vi "ProcessModbusUpdates.vi"(11 "MockFAILCSettings":T1={"ModbusRxDataFIFO"="ModbusSubnetARxDataFIFO", "ModbusTxDataFIFO"="ModbusSubnetATxDataFIFO", "BufferUpdateFIFO"="MockFAILC1Command", "Code17Memory"="MockFAILC1Code17", "Code18Memory"="MockFAILC1Code18", "Code65Memory"="MockFAILC1Code65", "Code72Memory"="MockFAILC1Code72", "Code74Memory"="MockFAILC1Code74", "Code75Memory"="MockFAILC1Code75", "Code76Memory"="MockFAILC1Code76", "Code80Memory"="MockFAILC1Code80", "Code110Memory"="MockFAILC1Code110", "Code120Memory"="MockFAILC1Code120", "Code121Memory"="MockFAILC1Code121", "CRCDataFIFO"="MockFAILC1CRCDataFIFO", "CRCCalculateFIFO"="MockFAILC1CRCCalculateFIFO", "CRCFIFO"="MockFAILC1CRCFIFO"}) -> ()   [LabVIEW 2016, in "FPGAMockFAILC.lvlib"]
uses:
  FPGAMockFAILC.lvlib
  DataTypes/MockFAILCSettings.ctl
  FPGAMockHPILC/DataTypes/MockHPModbusUpdateLoopData.ctl
  FPGAMockHPILC/DataTypes/MockHPModbusUpdateStates.ctl
  <vilib>/Platform/TimedLoop/XDataNode/timing_clust.ctl
  <vilib>/Platform/TimedLoop/XDataNode/nitl_modes.ctl
  <vilib>/Platform/TimedLoop/XDataNode/wakeup.ctl
  <vilib>/rvi/Emulation/niFpgaSctlEmulationGetInTimedLoop.vi
  <vilib>/rvi/Emulation/niFpgaEmulationReportErrorSimple.vi
  <vilib>/rvi/Emulation/niFpgaGetClockAttributes.vi
  <vilib>/rvi/Emulation/niFpgaCriticalErrorInLSC.vi
  <vilib>/rvi/DataTransferAndStorage/Container/Common/niFpgaContainerExecOnDevCompGetState.vi
  <vilib>/rvi/Emulation/niFpgaEmulationIsFPGAContextNoSignature.vi
  <vilib>/rvi/errors/niFpgaSetErrorForExecOnDevCompSimple.vi
  <vilib>/rvi/eio/common/nirviEmuReportErrorAndStop.vi
  <vilib>/rvi/DataTransferAndStorage/Container/Common/niFpgaContainerGetUniqueNameForEmu.vi
  <vilib>/rvi/FIFO/Fifo_Resource/nirvififoEmulationSetSize.vi
  <vilib>/rvi/FIFO/Fifo_Resource/nirviFifoEmulationQueueMgr.vi
  <instcachedir>/0/nirviFifoEmulationQueueMgr_E5CAEC123FF24DC58D834DCA3CDAA9B5.lvgen/nirviFifoEmulationQueueMgr_E5CAEC123FF24DC58D834DCA3CDAA9B5_002.vi
  <vilib>/rvi/FIFO/Fifo_Resource/nirvififoEmulationDetermineInputValidOut.vi
  <vilib>/rvi/FIFO/Fifo_Resource/nirvififoEmulationCreateLock.vi
  <vilib>/rvi/Emulation/niFpgaProcessEmulError.vi
  <vilib>/rvi/FIFO/Fifo_Resource/nirvififoEmulationObtainLock.vi
  <vilib>/rvi/FIFO/Fifo_Resource/nirvififoEmulationReleaseLock.vi
  <vilib>/rvi/occurrence/nirviWaitOnOccurrenceBase.vi
  <vilib>/rvi/errors/nirviReportUnexpectedCaseInternalError.vi
  <vilib>/rvi/errors/nirviReportUnexpectedCaseInternalError (U32).vi
  <vilib>/Utility/error.llb/Clear Errors.vi
  <vilib>/rvi/interface/RandomDataEmulation/niFpgaRandomDataHandleErrors.vi
  <instcachedir>/0/nirviFifoEmulationQueueMgr_E5CAEC123FF24DC58D834DCA3CDAA9B5.lvgen/nirviFifoEmulationQueueMgr_E5CAEC123FF24DC58D834DCA3CDAA9B5_000.vi
  <vilib>/rvi/Memory/Memory_Emulation/niFpgaMemoryEmulationCacheClearOnFirstRun.vi
  <vilib>/rvi/Memory/Memory_Emulation/nirvimemoryEmulationManagerCache_MakeExclusive.vi
  <vilib>/rvi/Memory/Memory_Emulation/niFpgaMemoryEmulationValidateCache.vi
  <vilib>/rvi/Memory/Memory_Emulation/nirvimemoryEmulationManagerCache_InsertValue.vi
  <vilib>/rvi/Memory/Memory_Emulation/nirvimemoryEmulationManagerCache_ReleaseExclusive.vi
  <vilib>/rvi/Memory/Memory_Emulation/nirvimemoryEmulationManagerCache_GetValue.vi
  <vilib>/rvi/Memory/Memory_Emulation/nirvimemoryEmulationManagerCache_SetValue.vi
  <vilib>/rvi/Emulation/niFpgaSctlEmulationResourceMgr.vi
  <instcachedir>/0/nirviFifoEmulationQueueMgr_E5CAEC123FF24DC58D834DCA3CDAA9B5.lvgen/nirviFifoEmulationQueueMgr_E5CAEC123FF24DC58D834DCA3CDAA9B5_001.vi
  <vilib>/Platform/TimedLoop/XDataNode/XDataNode.xnode
  <vilib>/rvi/DataTransferAndStorage/Container/XNode/niFpgaContainer.xnode
  <vilib>/rvi/FIFO/Fifo_Resource/niFpgaFifoEmulationRefIn.vi
  <vilib>/rvi/Memory/Memory_Emulation/niFpgaMemoryEmulationRefIn.vi
  FPGAMockHPILC/FPGAMockHPILC.lvlib
  <vilib>/Platform/TimedLoop/XDataNode/XDNodeRunTimeDep.lvlib
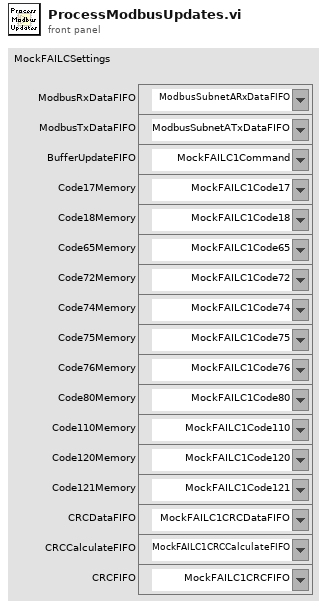
[diagram p1: front panel]
types:
  T1 = typedef "FPGAMockFAILC.lvlib/MockFAILCSettings.ctl" = cluster{"ModbusRxDataFIFO":refnum<k21>, "ModbusTxDataFIFO":refnum<k21>, "BufferUpdateFIFO":refnum<k21>, "Code17Memory":refnum<k21>, "Code18Memory":refnum<k21>, "Code65Memory":refnum<k21>, "Code72Memory":refnum<k21>, "Code74Memory":refnum<k21>, "Code75Memory":refnum<k21>, "Code76Memory":refnum<k21>, "Code80Memory":refnum<k21>, "Code110Memory":refnum<k21>, "Code120Memory":refnum<k21>, "Code121Memory":refnum<k21>, "CRCDataFIFO":refnum<k21>, "CRCCalculateFIFO":refnum<k21>, "CRCFIFO":refnum<k21>}
  T2 = typedef "FPGAMockHPILC.lvlib/MockHPModbusUpdateLoopData.ctl" = cluster{"ModbusUpdateLoopStates":T3, "Address":u32, "Function":u8, "ResponseLength":u32, "ResponseIndex":u32, "Index":u32, "Data":u16, "DelayTicks":u32}
  T3 = typedef "FPGAMockHPILC.lvlib/MockHPModbusUpdateStates.ctl" = enum16{"ReadModbusPort", "ProcessModbusData", "DelayMicroseconds", "WriteAddress", "WriteFunction", "WriteData", "WriteCRCLSB", "WriteCRCMSB", "WriteEndOfFrame", "CalculateCRC"}
  T4 = typedef "XDNodeRunTimeDep.lvlib/timing_clust.ctl" = cluster{"Expected End [f-1]":u64, "Actual End [f-1]":u64, "Finished Late? [f-1]":bool, "Expected End [i-1]":u64, "Actual End [i-1]":u64, "Finished Late? [i-1]":bool, "Expected Start [i]":u64, "Actual Start [i]":u64, "Expected Start [f]":u64, "Actual Start [f]":u64, "Source Name":string, "Structure Name":string, "Period":i64, "Deadline":i64, "Offset":i64, "Start":i64, "Priority":i32, "Timeout":i32, "Mode":T5, "Wakeup Reason":T6, "Error":errorcluster, "Source Type":string, "Secondary Source Type":string, "Global End Time":u64, "Global Start Time":u64, "Frame Duration":u64, "Iteration Duration":u64, "Assigned CPU":i32, "I/O Scan Engine Mode":u32}
  T5 = typedef "XDNodeRunTimeDep.lvlib/nitl_modes.ctl" = enum32{"No Change", "Process missed periods, maintain original phase", "Discard missed periods, maintain original phase", "Process missed periods, ignore original phase", "Discard missed periods, ignore original phase"}
  T6 = typedef "XDNodeRunTimeDep.lvlib/wakeup.ctl" = enum32{"Normal", "Aborted", "Asynchronous wakeup", "Timing source error", "Timed loop error", "Timeout"}
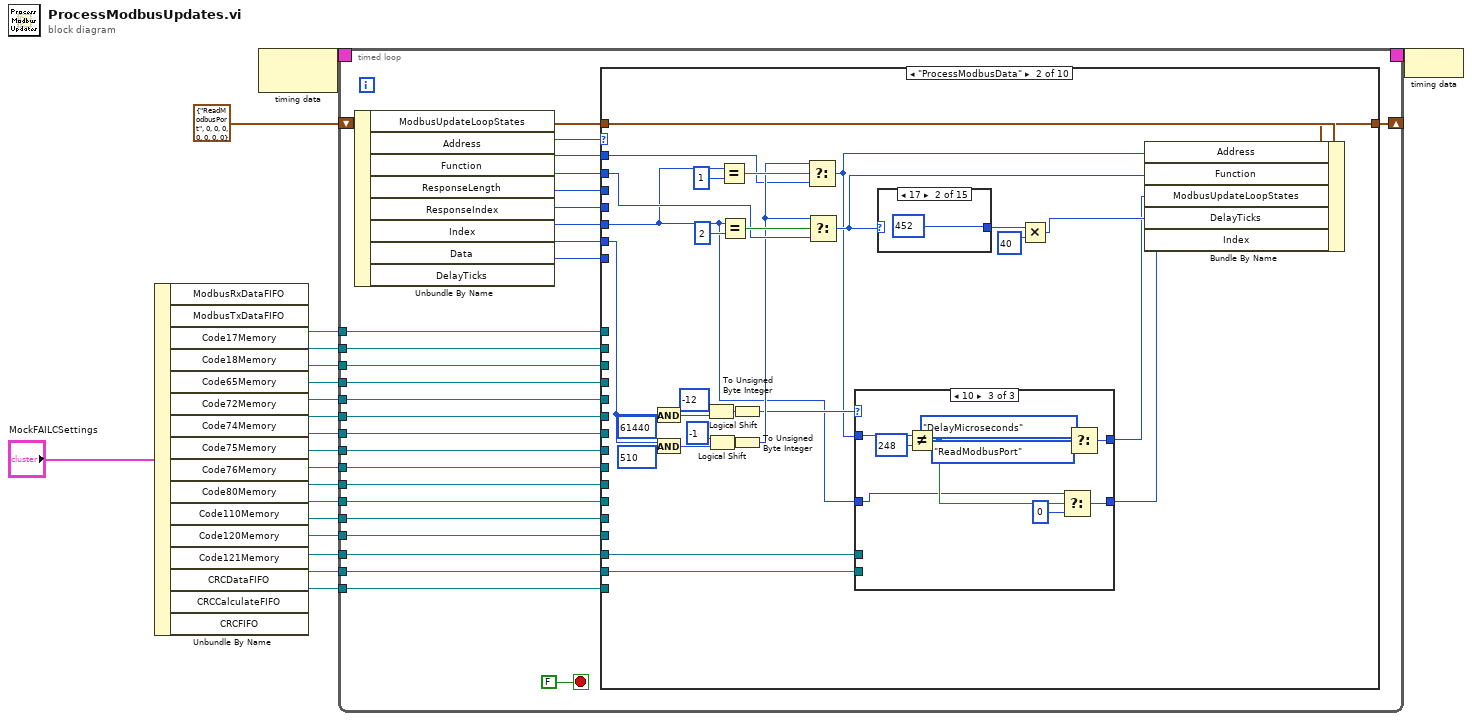
[diagram p0: block diagram]
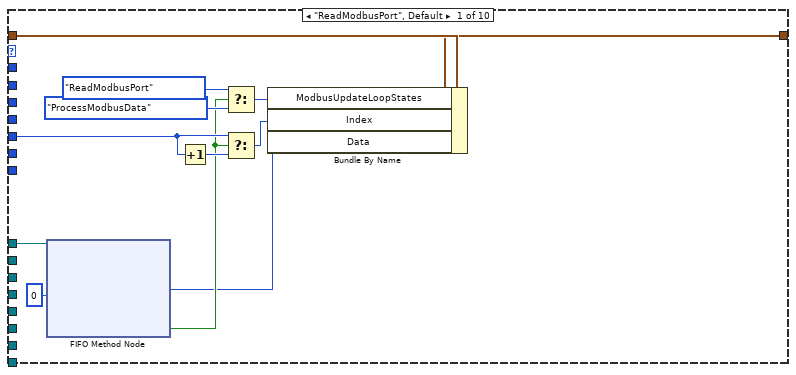
[diagram p2: hidden frame]
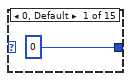
[diagram p3: hidden frame]
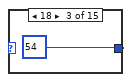
[diagram p4: hidden frame]
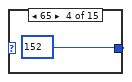
[diagram p5: hidden frame]
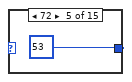
[diagram p6: hidden frame]
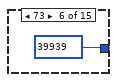
[diagram p7: hidden frame]
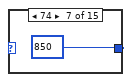
[diagram p8: hidden frame]
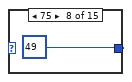
[diagram p9: hidden frame]
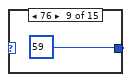
[diagram p10: hidden frame]
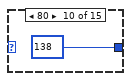
[diagram p11: hidden frame]
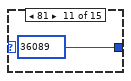
[diagram p12: hidden frame]
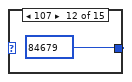
[diagram p13: hidden frame]
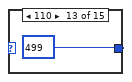
[diagram p14: hidden frame]
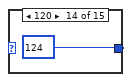
[diagram p15: hidden frame]
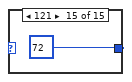
[diagram p16: hidden frame]
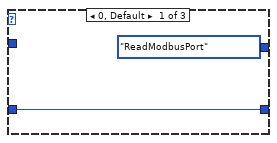
[diagram p17: hidden frame]
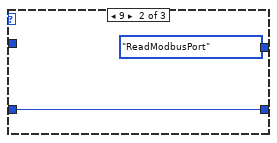
[diagram p18: hidden frame]
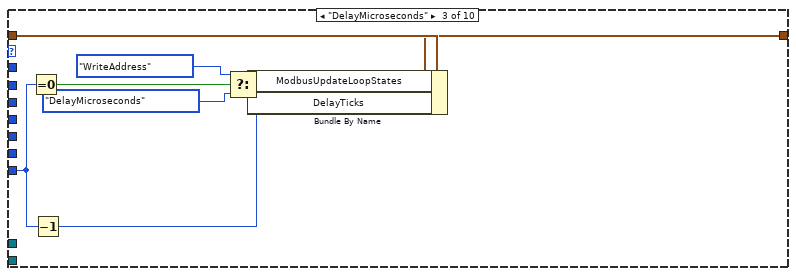
[diagram p19: hidden frame]
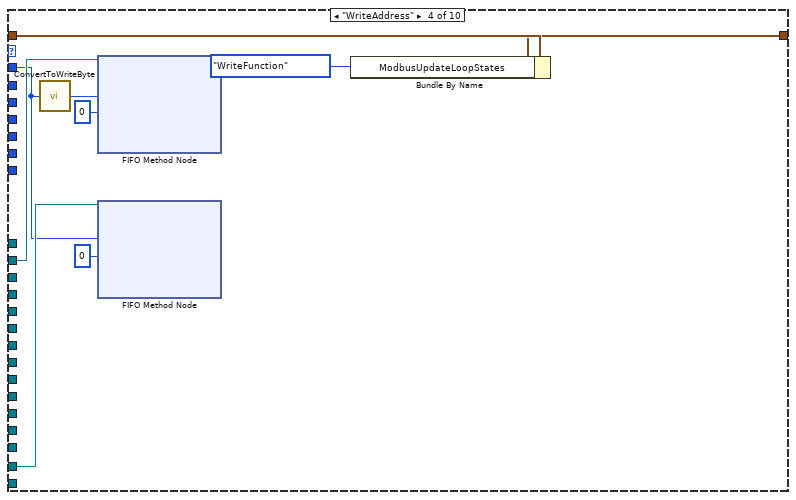
[diagram p20: hidden frame]
diagram:
  n1 = Unbundle By Name("MockFAILCSettings") -> ("ModbusRxDataFIFO"=w17:refnum<k21>, "ModbusTxDataFIFO"=w16:refnum<k21>, "Code17Memory"=w15:refnum<k21>, "Code18Memory"=w14:refnum<k21>, "Code65Memory"=w13:refnum<k21>, "Code72Memory"=w12:refnum<k21>, "Code74Memory"=w11:refnum<k21>, "Code75Memory"=w10:refnum<k21>, "Code76Memory"=w9:refnum<k21>, "Code80Memory"=w8:refnum<k21>, "Code110Memory"=w3:refnum<k21>, "Code120Memory"=w2:refnum<k21>, "Code121Memory"=w1:refnum<k21>, "CRCDataFIFO"=w7:refnum<k21>, "CRCCalculateFIFO"=w6:refnum<k21>, "CRCFIFO"=w5:refnum<k21>)
  n2 = node-c288() -> (w19:T4)  [unwired: 1 in]
  n3 = timed-loop {
    shift-right: [w42] -> _
    shift-left: T2 {"ModbusUpdateLoopStates"=enum."ReadModbusPort", "Address"=0, "Function"=0, "ResponseLength"=0, "ResponseIndex"=0, "Index"=0, "Data"=0, "DelayTicks"=0} ("MockHPBufferUpdateLoopData") -> [w41]
    timing: w19 -> [_]
    timing-out: [_] -> w18
    tunnel: w17 -> [w40]
    tunnel: w16 -> [w36]
    tunnel: w15 -> [w35]
    tunnel: w14 -> [w34]
    tunnel: w13 -> [w33]
    tunnel: w12 -> [w32]
    tunnel: w11 -> [w31]
    tunnel: w10 -> [w30]
    tunnel: w9 -> [w29]
    tunnel: w8 -> [w28]
    tunnel: w7 -> [w24]
    tunnel: w6 -> [w27]
    tunnel: w5 -> [w26]
    tunnel: w3 -> [w23]
    tunnel: w2 -> [w22]
    tunnel: w1 -> [w21]
    stop <- FALSE stop-if-true
    n4 = Unbundle By Name(w41) -> ("ModbusUpdateLoopStates"=w47:T3, "Address"=w46:u32, "Function"=w45:u8, "ResponseLength"=w44:u32, "ResponseIndex"=w43:u32, "Index"=w39:u32, "Data"=w38:u16, "DelayTicks"=w25:u32)
    n5 = case shown="\"ProcessModbusData\"" w47 {
      tunnel: w46 -> [_ w64 _ w126 _ w184 _ _ _ _]
      tunnel: w45 -> [_ w73 _ _ w135 w187 _ _ _ _]
      tunnel: w44 -> [_ _ _ _ _ w164 _ _ _ _]
      tunnel: w43 -> [_ _ _ _ _ w161 _ _ _ _]
      tunnel: [w50 w87 w123 w128 w139 w188 w254 w265 w279 w287] -> w42
      tunnel: w41 -> [w51 w88 w124 w130 w141 w189 w258 w266 w280 w292]
      tunnel: w40 -> [w59 _ _ _ _ _ _ _ _ _]
      tunnel: w39 -> [w54 w61 _ _ _ _ _ _ _ _]
      tunnel: w38 -> [_ w80 _ _ _ _ _ _ _ _]
      tunnel: w36 -> [_ _ _ w133 w144 w181 _ w260 w274 w291]
      tunnel: w35 -> [_ _ _ _ _ w186 _ _ _ _]
      tunnel: w34 -> [_ _ _ _ _ w180 _ _ _ _]
      tunnel: w33 -> [_ _ _ _ _ w179 _ _ _ _]
      tunnel: w32 -> [_ _ _ _ _ w178 _ _ _ _]
      tunnel: w31 -> [_ _ _ _ _ w177 _ _ _ _]
      tunnel: w30 -> [_ _ _ _ _ w176 _ _ _ _]
      tunnel: w29 -> [_ _ _ _ _ w175 _ _ _ _]
      tunnel: w28 -> [_ _ _ _ _ w174 _ _ _ _]
      tunnel: w24 -> [_ w77 _ w127 w136 w162 _ _ _ _]
      tunnel: w27 -> [_ w76 _ _ _ _ w257 _ _ _]
      tunnel: w26 -> [_ _ _ _ _ _ _ w264 w278 _]
      tunnel: w25 -> [_ _ w118 _ _ _ _ _ _ _]
      tunnel: w23 -> [_ _ _ _ _ w159 _ _ _ _]
      tunnel: w22 -> [_ _ _ _ _ w158 _ _ _ _]
      tunnel: w21 -> [_ _ _ _ _ w157 _ _ _ _]
      frame "ReadModbusPort", Default {
        n6 = xnode ("FIFO Method Node")("Timeout"=0, "FIFO In"=w59) -> ("Element"=w48:u16, "Timed Out?"=w49:bool)  [unwired: 1 out]
        n7 = Increment(x=w54) -> (x+1=w55:u32)
        n8 = Select(t=MockHPModbusUpdateStates."ReadModbusPort", s=w49, f=MockHPModbusUpdateStates."ProcessModbusData") -> (s? t:f=w53:T3)
        n9 = Select(t=w54, s=w49, f=w55) -> (s? t:f=w52:u32)
        n10 = Bundle By Name(cluster=w51, "ModbusUpdateLoopStates"=w53, "Index"=w52, "Data"=w48) -> (w50:T2)
      }
      frame "ProcessModbusData" {
        n11 = And(x=w80, y=u16 61440) -> (x .and. y?=w82:u16)
        n12 = And(x=w80, y=u16 510) -> (x .and. y?=w85:u16)
        n13 = Logical Shift(y=i16 -12, x=w82) -> (x << y=w70:u16)
        n14 = Logical Shift(y=i16 -1, x=w85) -> (x << y=w72:u16)
        n15 = Equal?(x=w61, y=u8 1) -> (x = y?=w78:bool)
        n16 = Equal?(x=w61, y=u8 2) -> (x = y?=w75:bool)
        n17 = To Unsigned Byte Integer(number=w70) -> (unsigned 8bit integer=w69:u8)
        n18 = To Unsigned Byte Integer(number=w72) -> (unsigned 8bit integer=w71:u8)
        n19 = Select(t=w71, s=w78, f=w64) -> (s? t:f=w63:u32)
        n20 = Select(t=w71, s=w75, f=w73) -> (s? t:f=w68:u8)
        n21 = case shown="10" w69 {
          tunnel: w77 -> [_ _ _]
          tunnel: w76 -> [_ _ _]
          tunnel: [MockHPModbusUpdateStates."ReadModbusPort" ("f") MockHPModbusUpdateStates."ReadModbusPort" ("f") w116] -> w62
          tunnel: w63 -> [_ _ w112]
          tunnel: w61 -> [w104 w106 w110]
          tunnel: [w104 w106 w108] -> w60
          frame 0, Default {
          }
          frame 9 {
          }
          frame 10 {
            n22 = Not Equal?(x=w112, y=u8 248) -> (x != y?=w111:bool)
            n23 = Select(t=w110, s=w111, f=u8 0) -> (s? t:f=w108:u32)
            n24 = Select(t=MockHPModbusUpdateStates."DelayMicroseconds" ("f"), s=w111, f=MockHPModbusUpdateStates."ReadModbusPort") -> (s? t:f=w116:T3)
          }
        }
        n25 = case shown="17" w68 {
          tunnel: [u32 0 ("Count(uSec)") u32 452 ("Count(uSec)") u32 54 ("Count(uSec)") u32 152 ("Count(uSec)") u32 53 ("Count(uSec)") u32 39939 ("Count(uSec)") u32 850 ("Count(uSec)") u32 49 ("Count(uSec)") u32 59 ("Count(uSec)") u32 138 ("Count(uSec)") u32 36089 ("Count(uSec)") u32 84679 ("Count(uSec)") u32 499 ("Count(uSec)") u32 124 ("Count(uSec)") u32 72 ("Count(uSec)")] -> w67
          frame 0, Default {
          }
          frame 17 {
          }
          frame 18 {
          }
          frame 65 {
          }
          frame 72 {
          }
          frame 73 {
          }
          frame 74 {
          }
          frame 75 {
          }
          frame 76 {
          }
          frame 80 {
          }
          frame 81 {
          }
          frame 107 {
          }
          frame 110 {
          }
          frame 120 {
          }
          frame 121 {
          }
        }
        n26 = Multiply(x=w67, y=u32 40) -> (x*y=w65:u32)
        n27 = Bundle By Name(cluster=w88, "Address"=w63, "Function"=w68, "ModbusUpdateLoopStates"=w62, "DelayTicks"=w65, "Index"=w60) -> (w87:T2)
      }
      frame "DelayMicroseconds" {
        n28 = Equal To 0?(x=w118) -> (x = 0?=w122:bool)
        n29 = Decrement(x=w118) -> (x-1=w117:u32)
        n30 = Select(t=MockHPModbusUpdateStates."WriteAddress", s=w122, f=MockHPModbusUpdateStates."DelayMicroseconds") -> (s? t:f=w121:T3)
        n31 = Bundle By Name(cluster=w124, "ModbusUpdateLoopStates"=w121, "DelayTicks"=w117) -> (w123:T2)
      }
      frame "WriteAddress" {
        n32 = call "ConvertToWriteByte.vi"("Input"=w126) -> ("Output"=w132:u16)
        n33 = xnode ("FIFO Method Node")("Element"=w132, "Timeout"=0, "FIFO In"=w133) -> ()  [unwired: 2 out]
        n34 = xnode ("FIFO Method Node")("Element"=w126, "Timeout"=0, "FIFO In"=w127) -> ()  [unwired: 2 out]
        n35 = Bundle By Name(cluster=w130, "ModbusUpdateLoopStates"=MockHPModbusUpdateStates."WriteFunction") -> (w128:T2)
      }
      frame "WriteFunction" {
        w137 = u8 0 ("ResponseIndex")
        n36 = call "ConvertToWriteByte.vi"("Input"=w135) -> ("Output"=w143:u16)
        n37 = case shown="121" w135 {
          tunnel: [u8 0 ("ResponseLength") u8 20 ("ResponseLength") u8 5 ("ResponseLength") u8 2 ("ResponseLength") u8 1 ("ResponseLength") u8 8 ("ResponseLength") u8 9 ("ResponseLength") u8 9 ("ResponseLength") u8 1 ("ResponseLength") u8 96 ("ResponseLength") u8 9 ("ResponseLength") u8 2 ("ResponseLength")] -> w138
          frame 0, Default {
          }
          frame 17 {
          }
          frame 18 {
          }
          frame 65 {
          }
          frame 72 {
          }
          frame 74 {
          }
          frame 75 {
          }
          frame 76 {
          }
          frame 80 {
          }
          frame 110 {
          }
          frame 120 {
          }
          frame 121 {
          }
        }
        n38 = xnode ("FIFO Method Node")("Element"=w143, "Timeout"=0, "FIFO In"=w144) -> ()  [unwired: 2 out]
        n39 = xnode ("FIFO Method Node")("Element"=w135, "Timeout"=0, "FIFO In"=w136) -> ()  [unwired: 2 out]
        n40 = Bundle By Name(cluster=w141, "ModbusUpdateLoopStates"=MockHPModbusUpdateStates."WriteData", "ResponseLength"=w138, "ResponseIndex"=w137, "Index"=w137) -> (w139:T2)
      }
      frame "WriteData" {
        n41 = Decrement(x=w184) -> (x-1=w185:u32)
        n42 = Multiply(x=w185, y=w164) -> (x*y=w183:u32)
        n43 = Add(x=w183, y=w161) -> (x+y=w182:u32)
        n44 = case shown="17" w187 {
          tunnel: w186 -> [_ w200 _ _ _ _ _ _ _ _ _ _]
          tunnel: w182 -> [_ w202 w207 w212 w217 w222 w227 w232 w237 w242 w247 w252]
          tunnel: [FALSE TRUE TRUE TRUE TRUE TRUE TRUE TRUE TRUE TRUE TRUE TRUE] -> w167
          tunnel: w180 -> [_ _ w205 _ _ _ _ _ _ _ _ _]
          tunnel: w179 -> [_ _ _ w210 _ _ _ _ _ _ _ _]
          tunnel: w178 -> [_ _ _ _ w215 _ _ _ _ _ _ _]
          tunnel: w177 -> [_ _ _ _ _ w220 _ _ _ _ _ _]
          tunnel: w176 -> [_ _ _ _ _ _ w225 _ _ _ _ _]
          tunnel: w175 -> [_ _ _ _ _ _ _ w230 _ _ _ _]
          tunnel: w174 -> [_ _ _ _ _ _ _ _ w235 _ _ _]
          tunnel: [u8 0 ("Data") w198 w203 w208 w213 w218 w223 w228 w233 w239 w244 w249] -> w160
          tunnel: w159 -> [_ _ _ _ _ _ _ _ _ w238 _ _]
          tunnel: w158 -> [_ _ _ _ _ _ _ _ _ _ w243 _]
          tunnel: w157 -> [_ _ _ _ _ _ _ _ _ _ _ w248]
          frame 0, Default {
          }
          frame 17 {
            n45 = xnode ("Memory Method Node")("Address"=w202, "Memory In"=w200) -> ("Data"=w199:u8)  [unwired: 1 out]
            n46 = feedback #1() -> (w198:u8)  [unwired: 1 in]
            n47 = feedback-in #1(w199) -> ()
          }
          frame 18 {
            n48 = xnode ("Memory Method Node")("Address"=w207, "Memory In"=w205) -> ("Data"=w204:u8)  [unwired: 1 out]
            n49 = feedback #2() -> (w203:u8)  [unwired: 1 in]
            n50 = feedback-in #2(w204) -> ()
          }
          frame 65 {
            n51 = xnode ("Memory Method Node")("Address"=w212, "Memory In"=w210) -> ("Data"=w209:u8)  [unwired: 1 out]
            n52 = feedback #3() -> (w208:u8)  [unwired: 1 in]
            n53 = feedback-in #3(w209) -> ()
          }
          frame 72 {
            n54 = xnode ("Memory Method Node")("Address"=w217, "Memory In"=w215) -> ("Data"=w214:u8)  [unwired: 1 out]
            n55 = feedback #4() -> (w213:u8)  [unwired: 1 in]
            n56 = feedback-in #4(w214) -> ()
          }
          frame 74 {
            n57 = xnode ("Memory Method Node")("Address"=w222, "Memory In"=w220) -> ("Data"=w219:u8)  [unwired: 1 out]
            n58 = feedback #5() -> (w218:u8)  [unwired: 1 in]
            n59 = feedback-in #5(w219) -> ()
          }
          frame 75 {
            n60 = xnode ("Memory Method Node")("Address"=w227, "Memory In"=w225) -> ("Data"=w224:u8)  [unwired: 1 out]
            n61 = feedback #6() -> (w223:u8)  [unwired: 1 in]
            n62 = feedback-in #6(w224) -> ()
          }
          frame 76 {
            n63 = xnode ("Memory Method Node")("Address"=w232, "Memory In"=w230) -> ("Data"=w229:u8)  [unwired: 1 out]
            n64 = feedback #7() -> (w228:u8)  [unwired: 1 in]
            n65 = feedback-in #7(w229) -> ()
          }
          frame 80 {
            n66 = xnode ("Memory Method Node")("Address"=w237, "Memory In"=w235) -> ("Data"=w234:u8)  [unwired: 1 out]
            n67 = feedback #8() -> (w233:u8)  [unwired: 1 in]
            n68 = feedback-in #8(w234) -> ()
          }
          frame 110 {
            n69 = xnode ("Memory Method Node")("Address"=w242, "Memory In"=w238) -> ("Data"=w240:u8)  [unwired: 1 out]
            n70 = feedback #9() -> (w239:u8)  [unwired: 1 in]
            n71 = feedback-in #9(w240) -> ()
          }
          frame 120 {
            n72 = xnode ("Memory Method Node")("Address"=w247, "Memory In"=w243) -> ("Data"=w245:u8)  [unwired: 1 out]
            n73 = feedback #10() -> (w244:u8)  [unwired: 1 in]
            n74 = feedback-in #10(w245) -> ()
          }
          frame 121 {
            n75 = xnode ("Memory Method Node")("Address"=w252, "Memory In"=w248) -> ("Data"=w250:u8)  [unwired: 1 out]
            n76 = feedback #11() -> (w249:u8)  [unwired: 1 in]
            n77 = feedback-in #11(w250) -> ()
          }
        }
        n78 = Increment(x=w161) -> (x+1=w169:u32)
        n79 = Increment(x=w164) -> (x+1=w163:u32)
        n80 = Equal To 0?(x=w161) -> (x = 0?=w168:bool)
        n81 = Equal?(x=w163, y=w169) -> (x = y?=w173:bool)
        n82 = Select(t=FALSE, s=w168, f=w167) -> (s? t:f=w166:bool)
        n83 = case shown="True" w166 {
          tunnel: w160 -> [_ w191]
          tunnel: w181 -> [_ w193]
          tunnel: w162 -> [_ w192]
          frame False {
          }
          frame True {
            n84 = call "ConvertToWriteByte.vi"("Input"=w191) -> ("Output"=w194:u16)
            n85 = xnode ("FIFO Method Node")("Element"=w194, "Timeout"=0, "FIFO In"=w193) -> ()  [unwired: 2 out]
            n86 = xnode ("FIFO Method Node")("Element"=w191, "Timeout"=0, "FIFO In"=w192) -> ()  [unwired: 2 out]
          }
        }
        n87 = Select(t=MockHPModbusUpdateStates."CalculateCRC", s=w173, f=MockHPModbusUpdateStates."WriteData") -> (s? t:f=w170:T3)
        n88 = Bundle By Name(cluster=w189, "ModbusUpdateLoopStates"=w170, "ResponseIndex"=w169) -> (w188:T2)
      }
      frame "CalculateCRC" {
        n89 = xnode ("FIFO Write")("Element"=TRUE, "Timeout"=0, "FIFO In"=w257) -> ()  [unwired: 2 out]
        n90 = Bundle By Name(cluster=w258, "ModbusUpdateLoopStates"=MockHPModbusUpdateStates."WriteCRCLSB") -> (w254:T2)
      }
      frame "WriteCRCLSB" {
        n91 = xnode ("FIFO Read")("Timeout"=0, "FIFO In"=w264) -> ("Element"=w261:u8, "Timed Out?"=w262:bool)  [unwired: 1 out]
        n92 = case shown="False" w262 {
          tunnel: w261 -> [w271 _]
          tunnel: w260 -> [w270 _]
          tunnel: [MockHPModbusUpdateStates."WriteCRCMSB" ("ModbusUpdateLoopStates") MockHPModbusUpdateStates."WriteCRCLSB" ("ModbusUpdateLoopStates")] -> w259
          frame False {
            n93 = call "ConvertToWriteByte.vi"("Input"=w271) -> ("Output"=w269:u16)
            n94 = xnode ("FIFO Write")("Element"=w269, "Timeout"=0, "FIFO In"=w270) -> ()  [unwired: 2 out]
          }
          frame True {
          }
        }
        n95 = Bundle By Name(cluster=w266, "ModbusUpdateLoopStates"=w259) -> (w265:T2)
      }
      frame "WriteCRCMSB" {
        n96 = xnode ("FIFO Read")("Timeout"=0, "FIFO In"=w278) -> ("Element"=w275:u8, "Timed Out?"=w276:bool)  [unwired: 1 out]
        n97 = case shown="False" w276 {
          tunnel: w275 -> [w285 _]
          tunnel: w274 -> [w284 _]
          tunnel: [MockHPModbusUpdateStates."WriteEndOfFrame" ("ModbusUpdateLoopStates") MockHPModbusUpdateStates."WriteCRCMSB" ("ModbusUpdateLoopStates")] -> w273
          frame False {
            n98 = call "ConvertToWriteByte.vi"("Input"=w285) -> ("Output"=w283:u16)
            n99 = xnode ("FIFO Write")("Element"=w283, "Timeout"=0, "FIFO In"=w284) -> ()  [unwired: 2 out]
          }
          frame True {
          }
        }
        n100 = Bundle By Name(cluster=w280, "ModbusUpdateLoopStates"=w273) -> (w279:T2)
      }
      frame "WriteEndOfFrame" {
        n101 = xnode ("FIFO Write")("Element"=u16 8416, "Timeout"=0, "FIFO In"=w291) -> ()  [unwired: 2 out]
        n102 = Bundle By Name(cluster=w292, "ModbusUpdateLoopStates"=MockHPModbusUpdateStates."ReadModbusPort") -> (w287:T2)
      }
    }
  }
  n103 = node-c288(w18) -> ()
